vi "Check if LogFile Exists.vi"(7 "Log File Path":path, 8 "error in (no error)":errorcluster, 11 "Target Information":T1) -> (0 "error out":errorcluster, 3 "Target Information out":T1, 5 "LogFile Exists?":bool)   [LabVIEW 2026, in "Telemetry System Tests.lvclass"]
uses:
  Telemetry System Tests.lvclass
  <vilib>/WebDAVClient/NI_WebDAV.lvlib
  <vilib>/NI/VeriStand Custom Device Testing Tools/VeriStandTestUtilities/ChassisInformation.ctl
  <vilib>/NI/VeriStand Custom Device Testing Tools/VeriStandTestUtilities/VeriStandTestUtilities.lvlib
  <vilib>/NI/VeriStand Custom Device Testing Tools/VeriStandTestUtilities/TargetInformation.ctl
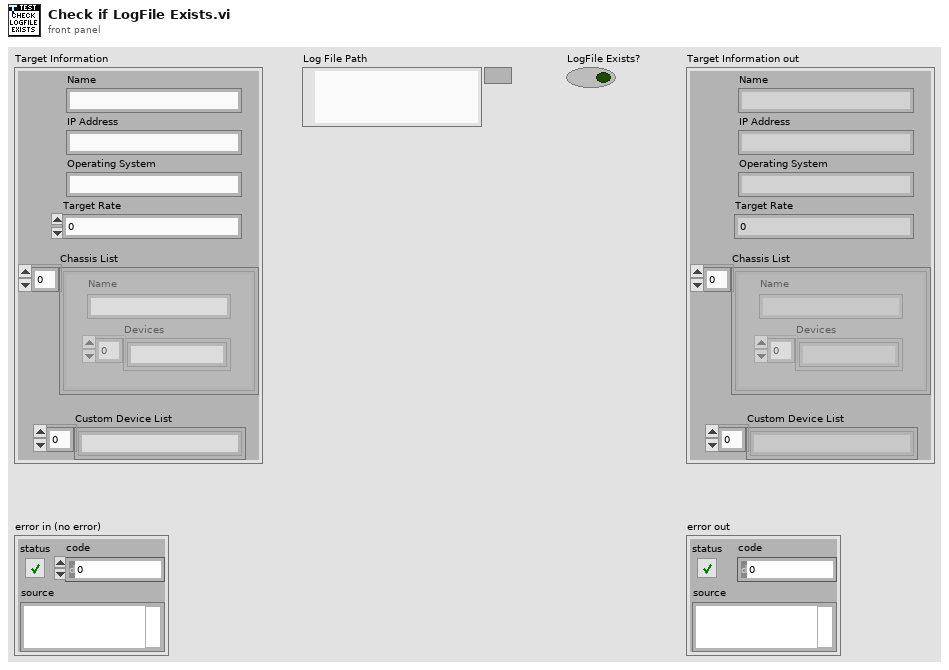
[diagram p1: front panel]
types:
  T1 = typedef "VeriStandTestUtilities.lvlib/TargetInformation.ctl" = cluster{"Name":string, "IP Address":string, "Operating System":string, "Target Rate":dbl, "Chassis List":T2[], "Custom Device List":string[]}
  T2 = typedef "VeriStandTestUtilities.lvlib/ChassisInformation.ctl" = cluster{"Name":string, "Devices":string[]}
  T3 = typedef "NI_WebDAV.lvlib/SessionHandle.ctl" = refnum<k1>
  T4 = typedef "NI_WebDAV.lvlib/FileInfo.ctl" = cluster{"type":string, "size":u64, "last modification":timestamp, "display name":string, "uri":string}
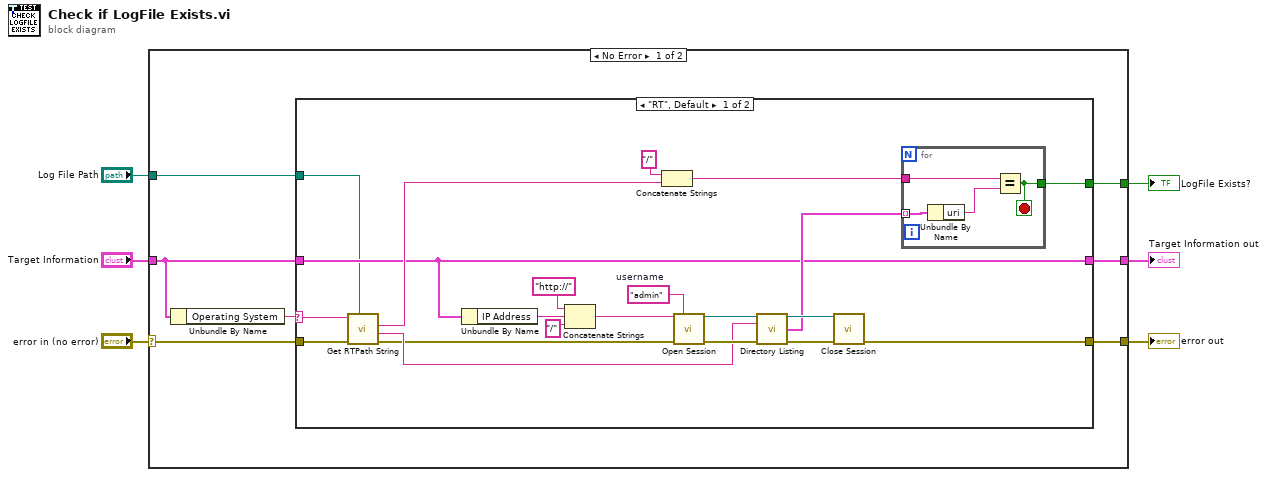
[diagram p0: block diagram]
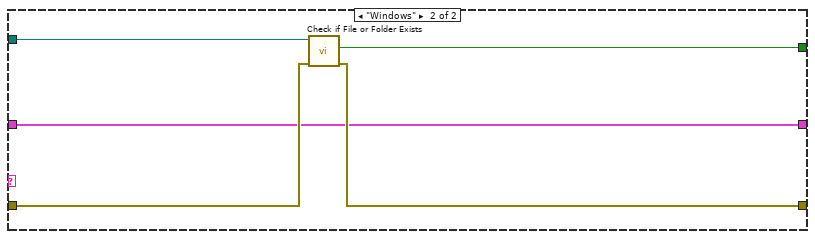
[diagram p2: hidden frame]
diagram:
  n1 = case shown="No Error" "error in (no error)" {
    selector: "error in (no error)" -> [w10 w45]
    tunnel: [w13 _] -> w6
    tunnel: "Log File Path" -> [w12 _]
    tunnel: [w11 w45] -> w4
    tunnel: "Target Information" -> [w7 w44]
    tunnel: [w8 w44] -> w1
    frame No Error {
      n2 = Unbundle By Name(w7) -> ("Operating System"=w9:string)
      n3 = case shown="\"RT\", Default" w9 {
        selector: w9 -> [w34 _]
        tunnel: [w27 w41] -> w11
        tunnel: w10 -> [w33 w42]
        tunnel: w12 -> [w15 w43]
        tunnel: [w19 w40] -> w13
        tunnel: w7 -> [w16 w39]
        tunnel: [w16 w39] -> w8
        frame "RT", Default {
          w14 = "admin"  # username
          n4 = call "Get RTPath String.vi"("SysDef Log File Path"=w15, "error in (no error)"=w33, "Target OS in"=w34) -> ("error out"=w17:errorcluster, "RT Folder Path"=w24:string, "RT File Path"=w22:string)  [unwired: 5 in, 1 out]
          n5 = Unbundle By Name(w16) -> ("IP Address"=w18:string)
          n6 = Concatenate Strings("http://" ("string"), w18, "/" ("string")) -> (w30:string)
          n7 = Concatenate Strings("/" ("string"), w22) -> (w21:string)
          n8 = call <vilib>:"Open Session.vi"("host uri prefix"=w30, "username"=w14, "error in (no error)"=w17) -> ("session handle out"=w28:T3, "error out"=w29:errorcluster)  [unwired: 11 in]
          n9 = call <vilib>:"Directory Listing.vi"("session handle"=w28, "relative uri"=w24, "error in (no error)"=w29) -> ("session handle out"=w26:T3, "file list"=w23:T4[], "error out"=w25:errorcluster)  [unwired: 9 in, 1 out]
          n10 = call <vilib>:"Close Session.vi"("session handle"=w26, "error in (no error)"=w25) -> ("error out"=w27:errorcluster)  [unwired: 13 in]
          n11 = for {
            tunnel: w23 -> [w38] mode=indexing
            tunnel: w21 -> [w36]
            tunnel: [w35] -> w19
            stop <- w35 stop-if-true
            n12 = Unbundle By Name(w38) -> ("uri"=w37:string)
            n13 = Equal?(x=w36, y=w37) -> (x = y?=w35:bool)
          }
        }
        frame "Windows" {
          n14 = call <vilib>:"Check if File or Folder Exists.vi"("error in (no error)"=w42, "path"=w43) -> ("error out"=w41:errorcluster, "file or folder exists?"=w40:bool)  [unwired: 7 in, 1 out]
        }
      }
    }
    frame Error {
    }
  }
  "LogFile Exists?" <- w6
  "error out" <- w4
  "Target Information out" <- w1
